vi "Untitled 1.vi"() -> ()   [LabVIEW 2023]
panel:
  out "output cluster":cluster{}
  out "index of element":i32
  out "safe mode starts":i32[](array[numeric])
  out "safe loop array":dbl[][](array[numeric])
  out "open loops starts":i32[](array[numeric])
  out "openloop array":dbl[][](array[numeric])
  out "safe start indexes":i32[](array[numeric])
  out "openloop start indexes":i32[](array[numeric])
  out "safemode indexdifference":i32[](array[numeric])
  out "openloop indexdifference":i32[](array[numeric])
  out "closed loop array":dbl[][](array[numeric])
  out "subarray 4":dbl[](array[numeric])
  out "subarray 3":dbl[](array[numeric])
  out "subarray 2":dbl[](array[numeric])
  out "closed loops starts":i32[](array[numeric])
  out "closed loop indexdifference":i32[](array[numeric])
  out "subarray":i32[](array[numeric])
  out "closed loop start indexes":i32[](array[numeric])
  out "element":i32
  out "closed loop indexes":i32[](array[numeric])
  out "size of  closedloop":i32
  out "closed index last element":i32
  out "open loop indexes":i32[](array[numeric])
  out "size of  openloop":i32
  out "ol index last element":i32
  out "open loop":dbl[](array[numeric])
  out "size of safe mode":i32
  out "safe mode indexes":i32[](array[numeric])
  out "closed loop const ref":dbl[](array[numeric])
  out "safe mode":dbl[](array[numeric])
  out "size of controllerstatereq":i32
  out "controllerstatereq":dbl[](array[numeric])
  in  "file path":path
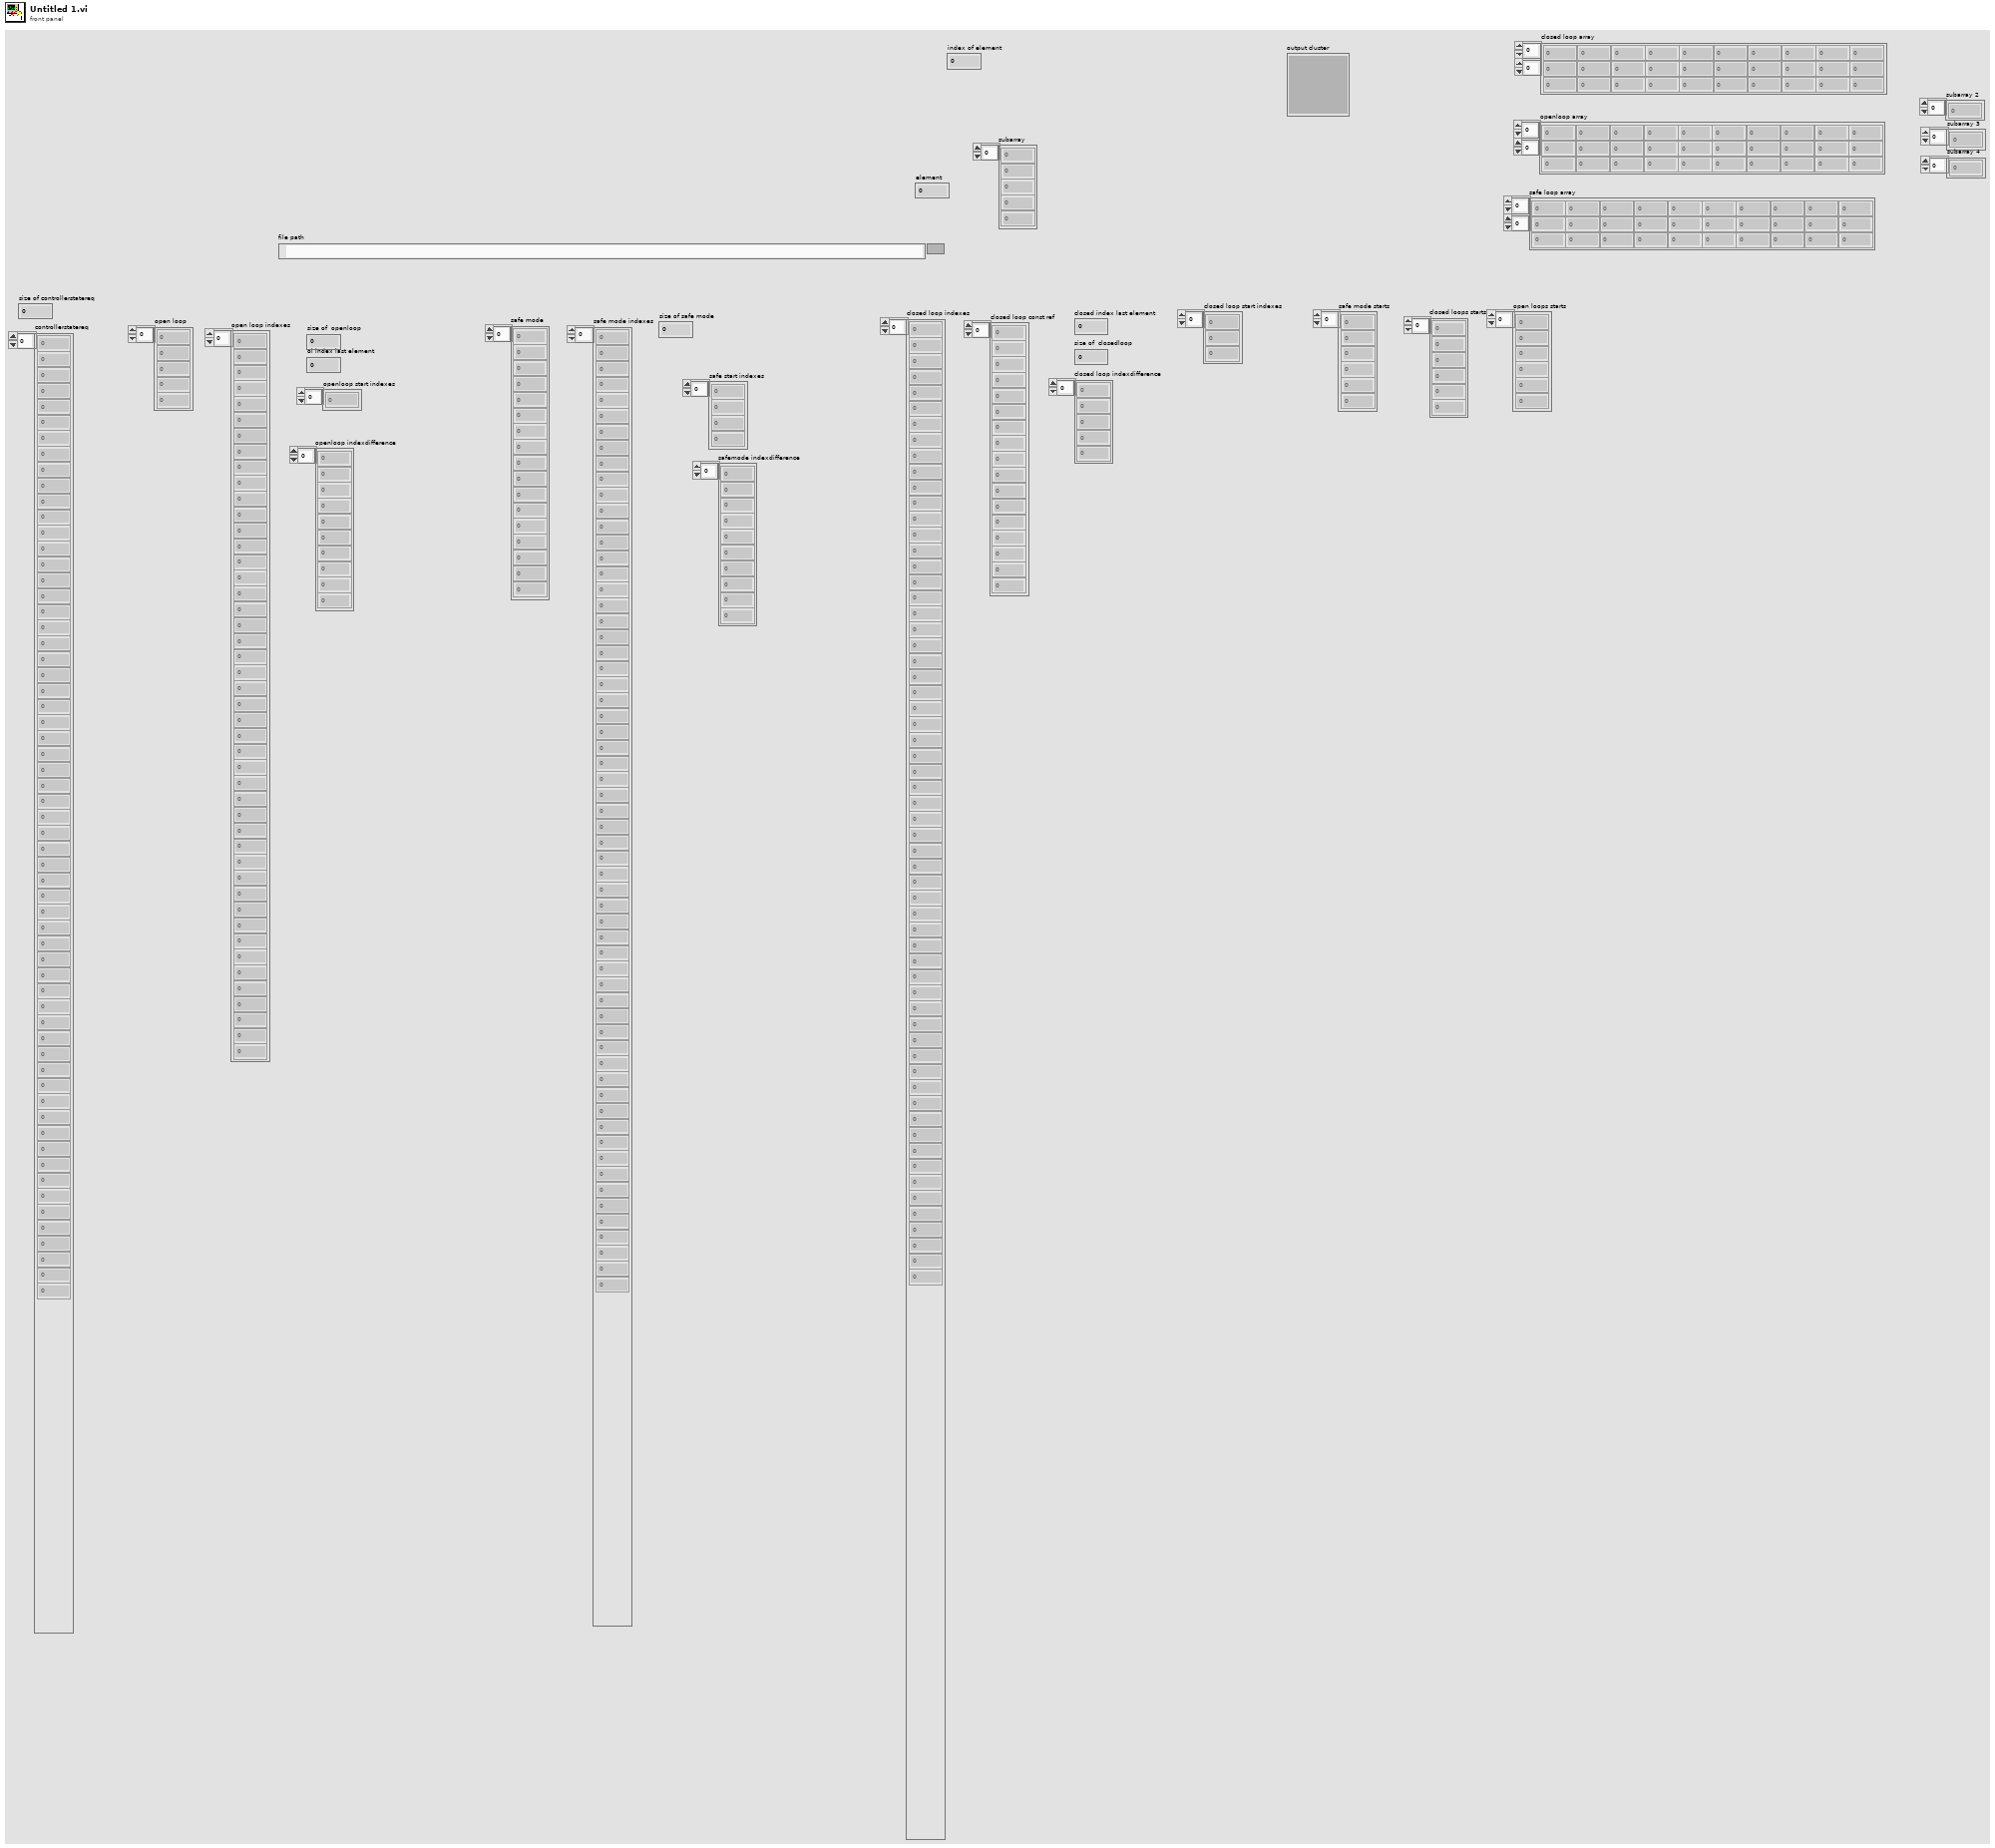
[diagram p1: front panel]
types:
  T1 = enum16{"open", "open or create", "create or replace", "create", "open (read-only)"}
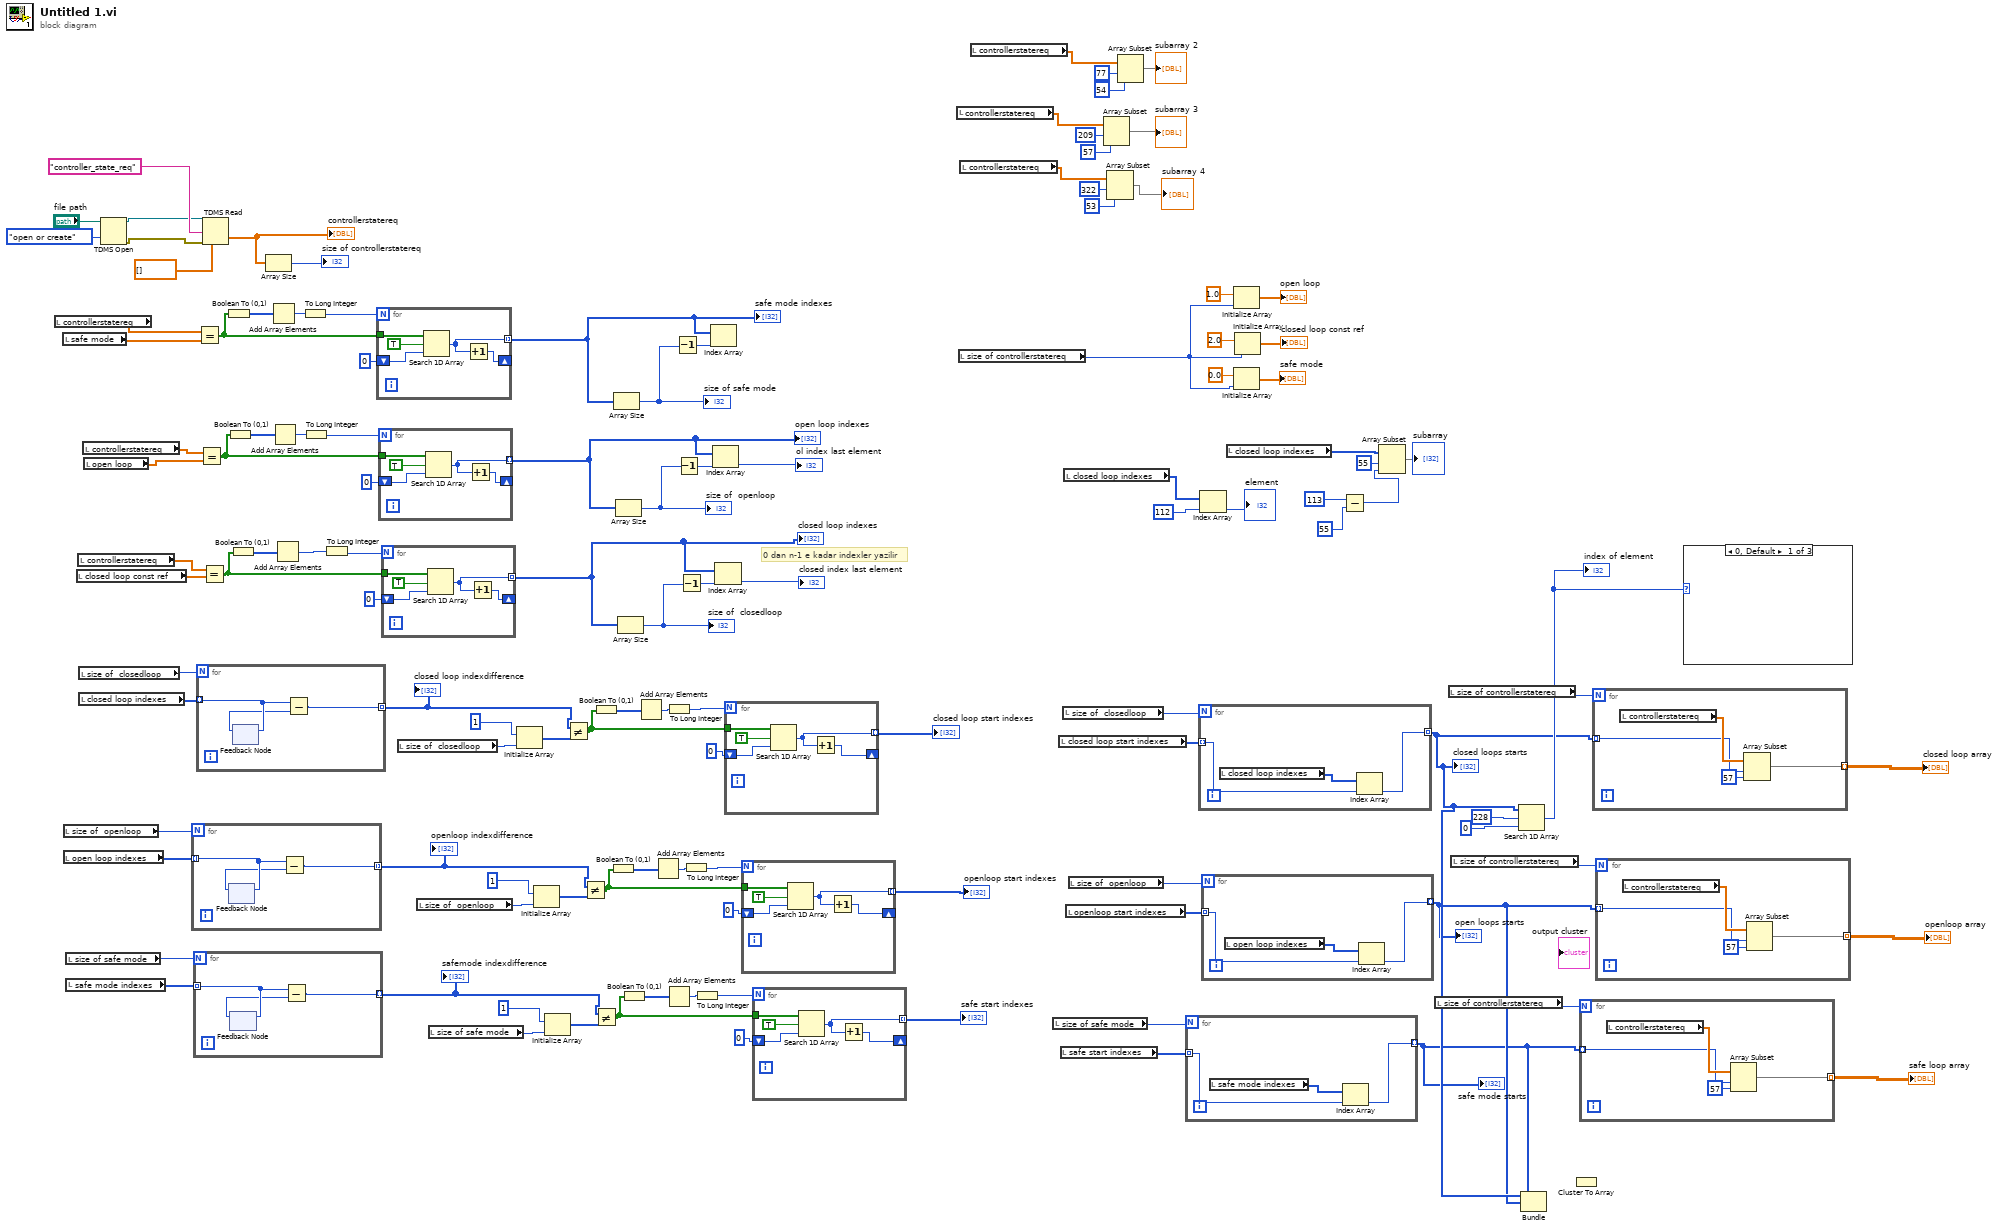
[diagram p0: block diagram]
diagram:
  # "0 dan n-1 e kadar indexler yazilir"
  n1 = local read "controllerstatereq"() -> (w110:dbl[])
  n2 = local read "safe mode"() -> (w109:dbl[])
  n3 = local read "size of  openloop"() -> (w39:i32)
  n4 = local read "open loop indexes"() -> (w38:i32[])
  n5 = local read "size of safe mode"() -> (w36:i32)
  n6 = local read "safe mode indexes"() -> (w37:i32[])
  n7 = local read "closed loop const ref"() -> (w82:dbl[])
  n8 = local read "controllerstatereq"() -> (w83:dbl[])
  n9 = local read "size of  closedloop"() -> (w60:i32)
  n10 = local read "closed loop indexes"() -> (w61:i32[])
  n11 = local read "controllerstatereq"() -> (w92:dbl[])
  n12 = local read "open loop"() -> (w91:dbl[])
  n13 = TDMS Open(10:T1."open or create" ("operation (0:open)"), 11:"file path") -> (0:w119:errorcluster, 3:w44:refnum<k34>)  [unwired: 5 in]
  n14 = for {
    N: w39 -> [_]
    tunnel: w38 -> [w125] mode=indexing
    tunnel: [w123] -> w27 mode=indexing
    n15 = feedback-in #1(w125) -> ()
    n16 = feedback #1() -> (w124:i32)  [unwired: 1 in]
    n17 = Subtract(x=w125, y=w124) -> (x-y=w123:i32)
  }
  "openloop indexdifference" <- w27
  n18 = for {
    N: w36 -> [_]
    tunnel: w37 -> [w128] mode=indexing
    tunnel: [w126] -> w18 mode=indexing
    n19 = feedback-in #2(w128) -> ()
    n20 = feedback #2() -> (w127:i32)  [unwired: 1 in]
    n21 = Subtract(x=w128, y=w127) -> (x-y=w126:i32)
  }
  "safemode indexdifference" <- w18
  n22 = for {
    N: w60 -> [_]
    tunnel: w61 -> [w131] mode=indexing
    tunnel: [w129] -> w41 mode=indexing
    n23 = feedback-in #3(w131) -> ()
    n24 = feedback #3() -> (w130:i32)  [unwired: 1 in]
    n25 = Subtract(x=w131, y=w130) -> (x-y=w129:i32)
  }
  "closed loop indexdifference" <- w41
  n26 = Equal?(x=w110, y=w109) -> (x = y?=w108:bool[])
  n27 = Equal?(x=w92, y=w91) -> (x = y?=w97:bool[])
  n28 = Equal?(x=w83, y=w82) -> (x = y?=w86:bool[])
  n29 = TDMS Read(0:w44, 7:"controller_state_req", 11:w119, 12:dbl[] []) -> (10:w67:dbl[])  [unwired: 4 in, 5 out]
  "controllerstatereq" <- w67
  n30 = Boolean To (0,1)(Boolean=w108) -> (0, 1=w114:i16[])
  n31 = Boolean To (0,1)(Boolean=w97) -> (0, 1=w93:i16[])
  n32 = Boolean To (0,1)(Boolean=w86) -> (0, 1=w90:i16[])
  n33 = Array Size(array=w67) -> (size(s)=→"size of controllerstatereq":i32)
  n34 = Add Array Elements(numeric array=w114) -> (sum=w111:i16)
  n35 = Add Array Elements(numeric array=w93) -> (sum=w96:i16)
  n36 = Add Array Elements(numeric array=w90) -> (sum=w87:i16)
  n37 = To Long Integer(number=w111) -> (32bit integer=w112:i32)
  n38 = To Long Integer(number=w96) -> (32bit integer=w95:i32)
  n39 = To Long Integer(number=w87) -> (32bit integer=w88:i32)
  n40 = for {
    N: w112 -> [_]
    tunnel: w108 -> [w132]
    shift-right: [w134] -> _
    shift-left: 0 ("start index (0)") -> [w133]
    tunnel: [w135] -> w107 mode=indexing
    n41 = Search 1D Array(1D array=w132, element=TRUE, start index (0)=w133) -> (index of element=w135:i32)
    n42 = Increment(x=w135) -> (x+1=w134:i32)
  }
  "safe mode indexes" <- w107
  n43 = for {
    N: w95 -> [_]
    tunnel: w97 -> [w137]
    shift-right: [w139] -> _
    shift-left: 0 ("start index (0)") -> [w138]
    tunnel: [w140] -> w98 mode=indexing
    n44 = Search 1D Array(1D array=w137, element=TRUE, start index (0)=w138) -> (index of element=w140:i32)
    n45 = Increment(x=w140) -> (x+1=w139:i32)
  }
  "open loop indexes" <- w98
  n46 = for {
    N: w88 -> [_]
    tunnel: w86 -> [w142]
    shift-right: [w144] -> _
    shift-left: 0 ("start index (0)") -> [w143]
    tunnel: [w145] -> w73 mode=indexing
    n47 = Search 1D Array(1D array=w142, element=TRUE, start index (0)=w143) -> (index of element=w145:i32)
    n48 = Increment(x=w145) -> (x+1=w144:i32)
  }
  "closed loop indexes" <- w73
  n49 = local read "size of  closedloop"() -> (w75:i32)
  n50 = local read "size of  openloop"() -> (w31:i32)
  n51 = local read "size of safe mode"() -> (w23:i32)
  n52 = Initialize Array(1, w75) -> (w66:i32[])
  n53 = Initialize Array(1, w31) -> (w34:i32[])
  n54 = Initialize Array(1, w23) -> (w20:i32[])
  n55 = Not Equal?(x=w41, y=w66) -> (x != y?=w65:bool[])
  n56 = Not Equal?(x=w27, y=w34) -> (x != y?=w35:bool[])
  n57 = Boolean To (0,1)(Boolean=w65) -> (0, 1=w78:i16[])
  n58 = Not Equal?(x=w18, y=w20) -> (x != y?=w19:bool[])
  n59 = Boolean To (0,1)(Boolean=w35) -> (0, 1=w28:i16[])
  n60 = Array Size(array=w107) -> (size(s)=w106:i32)
  "size of safe mode" <- w106
  n61 = Array Size(array=w98) -> (size(s)=w100:i32)
  "size of  openloop" <- w100
  n62 = Array Size(array=w73) -> (size(s)=w81:i32)
  "size of  closedloop" <- w81
  n63 = Boolean To (0,1)(Boolean=w19) -> (0, 1=w26:i16[])
  n64 = Add Array Elements(numeric array=w78) -> (sum=w76:i16)
  n65 = Add Array Elements(numeric array=w28) -> (sum=w30:i16)
  n66 = To Long Integer(number=w76) -> (32bit integer=w68:i32)
  n67 = Add Array Elements(numeric array=w26) -> (sum=w24:i16)
  n68 = Decrement(x=w106) -> (x-1=w105:i32)
  n69 = Decrement(x=w100) -> (x-1=w101:i32)
  n70 = Decrement(x=w81) -> (x-1=w84:i32)
  n71 = To Long Integer(number=w30) -> (32bit integer=w33:i32)
  n72 = To Long Integer(number=w24) -> (32bit integer=w21:i32)
  n73 = Index Array(array=w107, index=w105) -> ()  [unwired: 1 out]
  n74 = Index Array(array=w98, index=w101) -> (element=→"ol index last element":i32)
  n75 = Index Array(array=w73, index=w84) -> (element=→"closed index last element":i32)
  n76 = for {
    N: w68 -> [_]
    tunnel: w65 -> [w147]
    shift-right: [w149] -> _
    shift-left: 0 ("start index (0)") -> [w148]
    tunnel: [w150] -> w7 mode=indexing
    n77 = Search 1D Array(1D array=w147, element=TRUE, start index (0)=w148) -> (index of element=w150:i32)
    n78 = Increment(x=w150) -> (x+1=w149:i32)
  }
  "closed loop start indexes" <- w7
  n79 = for {
    N: w33 -> [_]
    tunnel: w35 -> [w152]
    shift-right: [w154] -> _
    shift-left: 0 ("start index (0)") -> [w153]
    tunnel: [w155] -> w9 mode=indexing
    n80 = Search 1D Array(1D array=w152, element=TRUE, start index (0)=w153) -> (index of element=w155:i32)
    n81 = Increment(x=w155) -> (x+1=w154:i32)
  }
  "openloop start indexes" <- w9
  n82 = for {
    N: w21 -> [_]
    tunnel: w19 -> [w157]
    shift-right: [w159] -> _
    shift-left: 0 ("start index (0)") -> [w158]
    tunnel: [w160] -> w8 mode=indexing
    n83 = Search 1D Array(1D array=w157, element=TRUE, start index (0)=w158) -> (index of element=w160:i32)
    n84 = Increment(x=w160) -> (x+1=w159:i32)
  }
  "safe start indexes" <- w8
  n85 = local read "controllerstatereq"() -> (w51:dbl[])
  n86 = local read "size of controllerstatereq"() -> (w102:i32)
  n87 = local read "controllerstatereq"() -> (w50:dbl[])
  n88 = local read "controllerstatereq"() -> (w56:dbl[])
  n89 = local read "size of safe mode"() -> (w12:i32)
  n90 = local read "closed loop start indexes"() -> (w59:i32[])
  n91 = local read "safe start indexes"() -> (w13:i32[])
  n92 = local read "size of  closedloop"() -> (w58:i32)
  n93 = local read "closed loop indexes"() -> (w64:i32[])
  n94 = local read "openloop start indexes"() -> (w14:i32[])
  n95 = local read "size of  openloop"() -> (w15:i32)
  n96 = Array Subset(array=w51, index=209, length=57 ("index")) -> (→"subarray 3":dbl[])
  n97 = Array Subset(array=w50, index=322, length=53 ("index")) -> (→"subarray 4":dbl[])
  n98 = Array Subset(array=w56, index=77, length=54 ("index")) -> (→"subarray 2":dbl[])
  n99 = for {
    N: w12 -> [_]
    tunnel: w13 -> [w163] mode=indexing
    tunnel: [w162] -> w1 mode=indexing
    n100 = local read "safe mode indexes"() -> (w164:i32[])
    n101 = Index Array(array=w164, index=w163) -> (element=w162:i32)
  }
  "safe mode starts" <- w1
  n102 = for {
    N: w58 -> [_]
    tunnel: w59 -> [w166] mode=indexing
    tunnel: [w165] -> w3 mode=indexing
    n103 = local read "closed loop indexes"() -> (w167:i32[])
    n104 = Index Array(array=w167, index=w166) -> (element=w165:i32)
  }
  "closed loops starts" <- w3
  n105 = Index Array(array=w64, index=112) -> (element=→"element":i32)
  n106 = for {
    N: w15 -> [_]
    tunnel: w14 -> [w169] mode=indexing
    tunnel: [w168] -> w2 mode=indexing
    n107 = local read "open loop indexes"() -> (w170:i32[])
    n108 = Index Array(array=w170, index=w169) -> (element=w168:i32)
  }
  "open loops starts" <- w2
  n109 = local read "closed loop indexes"() -> (w63:i32[])
  n110 = Initialize Array(1.0 ("element"), w102) -> (→"open loop":dbl[])
  n111 = Initialize Array(0.0 ("element"), w102) -> (→"safe mode":dbl[])
  n112 = Initialize Array(2.0 ("element"), w102) -> (→"closed loop const ref":dbl[])
  n113 = Subtract(x=113 ("index"), y=55 ("index")) -> (x-y=w69:i32)
  n114 = Array Subset(array=w63, index=55, length=w69) -> (→"subarray":i32[])
  n115 = local read "size of controllerstatereq"() -> (w11:i32)
  n116 = local read "size of controllerstatereq"() -> (w57:i32)
  n117 = local read "size of controllerstatereq"() -> (w16:i32)
  n118 = Search 1D Array(1D array=w3, element=228, start index (0)=0) -> (index of element=w4:i32)
  "index of element" <- w4
  n119 = Bundle(w3, w2, w1) -> ()  [unwired: 1 in, 1 out]
  n120 = Cluster To Array() -> ()  [unwired: 1 in, 1 out]
  n121 = for {
    N: w11 -> [_]
    tunnel: w1 -> [w173] mode=indexing
    tunnel: [w172] -> w10 mode=indexing
    n122 = local read "controllerstatereq"() -> (w174:dbl[])
    n123 = Array Subset(array=w174, index=w173, length=57) -> (w172:dbl[])
  }
  "safe loop array" <- w10
  n124 = for {
    N: w57 -> [_]
    tunnel: w3 -> [w177] mode=indexing
    tunnel: [w176] -> w40 mode=indexing
    n125 = local read "controllerstatereq"() -> (w178:dbl[])
    n126 = Array Subset(array=w178, index=w177, length=57) -> (w176:dbl[])
  }
  "closed loop array" <- w40
  n127 = for {
    N: w16 -> [_]
    tunnel: w2 -> [w181] mode=indexing
    tunnel: [w180] -> w17 mode=indexing
    n128 = local read "controllerstatereq"() -> (w182:dbl[])
    n129 = Array Subset(array=w182, index=w181, length=57) -> (w180:dbl[])
  }
  "openloop array" <- w17
  n130 = case shown="0, Default" w4 {
    frame 0, Default {
    }
    frame 1 {
    }
    frame 2 {
    }
  }
